vi "Main_16B_X1.vi"() -> ()   [LabVIEW 2024]
uses:
  Cluster_Deer Score and Pose and Set.ctl
  Cluster_Deer Pose.ctl
  Utility/Universal Utility/TypeDefs_Utility/Cluster_Row-Column.ctl
  Utility/Universal Utility/TypeDefs_Utility/ENUM_4 Directions U-D-L-R.ctl
  8beb7c92-1c82-4182-b844-b29be1e81950.vi
  <vilib>/Utility/error.llb/Trim Whitespace.vi
  <vilib>/Utility/error.llb/Trim Whitespace One-Sided.vi
panel:
  out "size(s)":i32
  out "Answer":i32
  out "sorted array":T1[](array[typedef])
  in  "Tab Control":enum32{"Example ", "Eample 2", "Puzzle"}(tab)
  in  "Example":string="###############\n#.......#....E#\n#.#.###.#.###.#\n#.....#.#...#.#\n#.###.#####.#.#\n#.#.#.......#.#\n#.#.#####.###.#\n#...........#.#\n###.#.#####.#.#\n#...#.....#.#.#\n#.#.#.###.#.#.#\n#.....#...#.#.#\n#.###.#.#.#.#.#\n#S..#.....#...#\n###############"
  in  "Example 2":string="#################\n#...#...#...#..E#\n#.#.#.#.#.#.#.#.#\n#.#.#.#...#...#.#\n#.#.#.#.###.#.#.#\n#...#.#.#.....#.#\n#.#.#.#.#.#####.#\n#.#...#.#.#.....#\n#.#.#####.#.###.#\n#.#.#.......#...#\n#.#.###.#####.###\n#.#.#...#.....#.#\n#.#.#.#####.###.#\n#.#.#.........#.#\n#.#.#.#########.#\n#S#.............#\n#################"
  in  "Puzzle":string="#############################################################################################################################################\n#.....#.....#.....#.........#.....#.......#...#.........#.....#.....#...........#...#.............#.....#.....#...........#.....#..........E#\n#.###.#.###.#.###.#####.#.#.#.###.#.#####.#.#.#.###.###.#.#.###.###.#.#######.###.#.#.###.#######.###.#.###.###.###.#####.#.###.#.#####.###.#\n#.#.....#.#.#.#.....................#.....#.....#...#...#.#.......#.#...#...#.....#.#.#.#.....#.#.....#...#...#.#.#...#.....#...#...#...#...#\n#.#######.#.#.#######.###.#.###.###.#.#.###.#####.#.#.###.#######.#.###.#.#.#######.#.#.#####.#.#########.###.#.#.###.#######.###.###.###.###\n#...........................#...#...#.#.#...........#.#...#.#...#.#.#...#.#.....#...........................#.......#...#...#...#.#...#.....#\n#.###.#.#.#.###.#.#.#######.#####.#.#.#.#.###.###.#.#.#.###.#.#.###.#.###.#####.#.#.#####.#.###.###.#######.###########.#.#.###.#.#.###.#####\n#.#...#.#.#.#...#.#...#...........#.........................#.#...#.#.#...#...#.#.#...#...#.#.......#.#...#.........#...#.#.#...#.#.#...#...#\n#.#.###.#.#.#.###.#####.#####.#####.#.###.###.#.#.#.#########.###.#.#.#####.#.#.#.###.#.###.#.#######.#.#.#########.#.#####.#.###.#.#####.#.#\n#.#...#.#...#.#.......#.#.....#...#.#...#.....#...#...........#.#.#.........#...#...............................#...#...#...#.#...#...#...#.#\n#.###.#.#####.#######.#.#.#######.#.#.#.#######.#.#.#.###.#####.#.###.#.#######.#######.#.#.#####.###.#.#.#.#.#.#.#####.#.###.#######.#.###.#\n#.#.#.#.......#.......#...#.#.....#.#.#.......#.#.#.#.#...#...#.....#.#.....#...#.........#.#...#.....#.................#.......#...#...#...#\n#.#.#.#########.#####.#####.#.#.###.#.#.#######.#.#.#.#.###.#.#####.#.#####.#.#########.#.#.###.###.###.#.#.###.#.#.#.#########.#.#.#####.#.#\n#...#.#.........#.......#...#.#.....#.#.....#...#...........................#.........#...#.............#.#...#...#.#.....#...#...#.......#.#\n###.#.#.#####.###.###.#.#.#.#.#######.#####.#.###.###.###.#.#####.#.#.###########.###.#.#####.#.#.###.###.###.#####.#####.#.#.#############.#\n#...#.#.....#.....#...#...#.......#.....#...#.#.....#.#...#.#...#.#...#.............#.#...#...#.....#...#...#.#...#.#...#...#.#.............#\n#.#.#.#####.#######.#.###########.#.#####.#.#.#.###.#.#####.#.###.###.#######.#.#.###.###.#.#######.#.#####.#.#.#.#.#.#.#####.###.#.#######.#\n#...#...#.#...#.....#.........#...#...#...#.#.#.#...#.......#...#.#.#.#.....#.#...#.......#.......#.#.#.....#.#.#.....#.....#...#.#.....#...#\n#.#####.#.###.#####.#########.#.###.#.#.###.#.###.#############.#.#.#.#.###.#.#.###.###########.#.#.#.#.#####.#.###########.###.#####.#.#.###\n#.#.....#...#.....#.........#...#.#...#...#.#...#...#...........#.#...#.#.#.#.#.....#.#.......#.#.....#.#...#.#...#...#.....#.#.....#.#...#.#\n#.#.#.#####.###.#.#####.#########.###.###.#.###.#.#.#.###.#####.#.#.###.#.#.#####.###.#.#####.#########.#.#.#.#.###.#.#.#####.#####.#.#####.#\n#.#.#.#...#.....#.....#...............#...#.#.#.#...#.#.#...#.#.#.#.#...#.#.....#.....#.#...#.....#.....#.#.#.#.#...#.#.#.....#.....#.#.....#\n#.#.###.#.#.#########.#.###############.###.#.#.#.###.#.###.#.#.#.#.#.###.#####.#######.#.#######.#.#######.#.###.###.#.#.#.###.#####.#.###.#\n#.#.....#.#.......#...#...#...........#...#...#.#...#.#...#.#.#.#.#...#.........#.......#.......#.#.#.......#.....#.#.#.#.#.#.......#.#.#...#\n#.#######.#####.###.#####.#.#.#######.###.#####.###.#.#.#.#.#.#.#.#############.#.#########.###.#.#.###.###########.#.#.#.###.###.#.#.#.###.#\n#.#.....#.#...#.#...#...#.#.#.#.....#.#.#.....#...#.....#...#.#.#...#.........#...........#...#.....#...#.........#...#.#...#.#...#.#.#...#.#\n#.#.#####.#.#.#.#.###.###.###.#.###.#.#.#####.###.###.#####.#.#.###.#.#######.#.#######.#.###########.###.#######.#.###.#.#.#.###.###.###.#.#\n#...#.....#.#...#...#...#.....#...#.........#.......#.#...#.#.....#.........#.#.#.....#.#.......#.....#.....#...#.#.#...#.#.#...#...#.....#.#\n###.#.#####.###.###.###.#.###############.#######.#.###.#.#.#.#############.#.#.#.###.#########.#.#####.#####.#.#.#.###.###.###.#.#.#######.#\n#.#.#.#.......#.#.#...#...#.............#.#.......#...#.#...#.#...........#.#.#...#.#...........#.........#...#...#...#.....#...#...........#\n#.#.#.#.#.#.#.#.#.###.#.#.#.#####.#.###.###.#####.###.#.#####.#.#.#######.###.#.###.#############.#########.#.#######.#.#####.###.#.###.#####\n#...#.#.#...#.#.....#.#...#.......#.#...#...#...#...#...#...#.#...#.....#.#...#...........#.....#...#.......#.#.....#...#.....#...#...#.#...#\n#.###.#.#####.###.###.#.#######.#.#.#.###.###.#####.#####.###.#.#.#.###.#.#.###.###.#######.###.###.#.#######.#.###.#.#.#.###.#####.#.#.###.#\n#...#.#.#...#.#.#.#...#...#.#...#...#.#...#...........#.....#...#.#...#.#...#...#.#.#.......#.#...#.#.......#.....#...#.#...#.#.....#.#...#.#\n###.#.###.#.#.#.#.#.#####.#.#.#######.#.###.#########.#####.###.#.###.#.#####.###.#.#.#######.###.#.#######.#####.#########.###.###.#.###.#.#\n#...#.#...#...#...#...#.....#...#...#.#...#.....#...#.....#.....#...#.#...#.......#.#.....#...#...#.#.....#.......#...........#...#.#.......#\n#####.#.#.###.#######.#.#######.#.###.#.#.#######.#.#####.#######.#.###.#.#.#######.#####.#.#.#.###.#####.#########.#.###.#.#.#.###.#######.#\n#...#.#.#.....#...#...#.#.......#.....#.#.......#.#...#...#.....#.#...#.#.#...........#.#.#.#.#...#.#.....#...#.....#.#.#.#.#.......#...#...#\n#.#.#.#.#.#####.#.#.#####.###.###.#####.#.#####.#.###.###.#.###.#####.#.#####.#.#####.#.#.###.###.#.#.###.###.#.###.#.#.#.#######.#.#.#.#.###\n#...............#.........#...........#.#.....#.#...#...#...#...#.....#.......#.#...#.#.#...#...#.....#...#...#.#.....#.#...#.....#...#.#...#\n#.#####.#.#################.#########.###.###.#.###.###.#####.###.###.#.#.#####.#.#.#.#.###.#.#.#####.#.###.#.#.#.#####.###.#.###.#.###.###.#\n#...#.#...#...#...#.....#...#.......#...#...#...#...#.#.....#.#...#.#.........#.#...#.......#.#.......#.#...#.#.#.........#.#.............#.#\n###.#.###.#.#.#.#.###.###.###.#####.###.###.###.#.###.#####.#.#.###.#.#.#######.#.###.#####.###.#######.###.###.#.#####.###.#.#####.#.###.#.#\n#...#...#...#.#.#...#.......#.#...#.#...#.....#.#.#...#.....#...#.....#.........#.....#.....#...#.....#...#.....#.....#.....#.#.......#.#.#.#\n#.###.#.#.###.#.###.#.#.#####.#.#.#.###.#.#.#.#.#.#.#.#.#########.#####.#########.#####.#####.###.###.###.#.#########.#.#####.#.###.###.#.###\n#...#.#.......#...#...#.#.....#.#.#...#...#.....#.#.#.#.#...#.......#...#.........#.....#.....#...#.#...#.#.......#.#.#...#.....#.......#...#\n#.#.#####.#.#.#.#.###.###.#####.#.###.#####.#####.#.#.#.#.###.#######.###.###.#.###.#######.#.#.###.###.#.#######.#.#.###.#.#######.#.#.###.#\n#.#.......#...#...#.#...#.....#.....#.#...#...#...#.#.#.#.....#.......#...#...#...#.#.......#...#.....#...#.#.......#.#...#.#.......#.#.#.#.#\n#.#######.###.#.###.###.#####.#.###.#.#.#.###.#.#####.#.#######.###########.#.#####.###.#####.#.#.#.#######.#.#####.#.#.###.#####.#.#.#.#.#.#\n#.....#.#.............#.#...#...#...#.#.#...#.#...#...#.#.....#...#...#...#...#...#.....#.....#.#.#.#...#...#.#...#.#.#.#...#.....#.#.#...#.#\n#.###.#.#.###.#######.#.#.#.#.#.#####.#.###.#.###.#.#.#.#.###.###.#.#.#.#.#.#.#.#.#######.#####.#.###.#.#.#.#.#.#.###.#.#.#.#.#####.#.#####.#\n#.............#...#...#...#.....#.....#...#.........#.#...#.#.#...#.#...#...#...#...#.....#.....#.....#...#.#.#.#...#.#...#...#...#...#.....#\n#.###########.#.#.###############.#######.#############.###.#.#.#.#.###############.#.#.#.#.#####.#########.#.#.#.#.#.###.#####.###.#.#.###.#\n#.#.....#.....#.#...........#...#.......#.#...#.......#.....#.#.#.#.#...#.....#...#...#.#.#.....#.........#...#.#.#...#.........#.....#.#.#.#\n###.###.#.#.#.#.###.#######.#.#.#######.#.#.###.#####.#####.#.#.#.#.###.#.#.#.#.#.#####.#.#####.#########.#####.#.#####.###.###.#.#####.#.#.#\n#...#...#.#.....#.......#.#...#...#...#.#.....#.#...#.....#.#.#.#.#...#.#.#.#...#.#...#.#.#.....#...#...........#...#...#.....#.#.#.....#.#.#\n#.#####.#.###.###.#####.#.#######.#.#.#.#.#.#.#.#.#.#####.###.#.#####.#.#.#.#####.###.#.#.#.#####.#.#######.#######.#.###.#####.#.#.#####.#.#\n#.....#.#.......#.#...#.....#...#...#.#.#.#...#.#.#.....#...#.#.......#...#.#.........#.#.#.#.....#...#...#.#.....#...#...#...#...#...#.#...#\n#.###.#.#######.#.#.#.#.#####.#.###.#.#.#.#.###.#.#####.#.#.#.###.#########.#.#######.#.#.#.###.#.###.#.#.#.#.###.#.#####.#.#.#.#####.#.#.###\n#...#.#.#...#...#.#.#...#...#.#.............#...#.#...#.....#...#...........#...#.....#.#.#...#.#...#...#.#.....#.#.#...#.#.#.#.....#.#.....#\n#####.#.#.#.#.###.#######.#.#.#############.#.###.###.#########.###############.#.#####.#.###.#.###.###.#.#####.#.#.#.#.###.#.###.###.#####.#\n#.....#...#.#.#.#.........#...#.#...#.......#...#...#.....#.....#.........#...#.#.#.....#.#...#.#...#...#...#.#.#.#...#.....#...#.#...#...#.#\n#.#####.###.#.#.#.#.###########.#.#.#.#########.###.#.###.#.#.###.#######.#.#.#.#.#.#####.#.#####.###.#.###.#.#.#.#############.#.#.#.#.#.#.#\n#.............#.#.....#.........#.#...#.....#.#...#...#.#.#.#...#...#...#...#.#.........#.#.......#.........#...#.....#.........#.#.#.#.#.#.#\n#.###########.#.#####.###.#####.#.#####.#.#.#.###.#####.#.#.###.#.###.#.#.###.#.#######.#######.#.#########.#.#######.#########.###.###.#.#.#\n#.#.......#...#.....#.#...#.#...#.#...#.#.......#.#...#...#.#...#.#...#.#.#...#.#.....#.......#.#.#...#...#.#.......#...#.....#.....#...#.#.#\n#.#.#####.#.#.#.#.#.#.#.###.#.#.#.#.#.#.#.#.#####.#.#.#.#####.###.#.###.###.###.###.#####.#####.#.#.#.#.#.#.###########.#.###.#.#####.###.#.#\n#...#...#.#.#.#.#.#.#.#.#.......#...#.#.#.#.#.....#.#.#.......#...#.#.....#.#.......#.....#.....#...#...#.#...........#...#...#.#.....#.#.#.#\n#.###.#.#.###.#.#.###.#.#.###########.#.#.###.#####.#.#######.#.###.#####.#.#########.###.#.#########.###.###########.###.#.###.#.#####.#.###\n#.....#.#...#...#.....#.#.#.........#.#.#.#...#.....#.....#...#.........#.#.........#...#...........#...#.#.........#...#.#.#.#.#.#.........#\n#######.###.#.#####.###.###.#######.#.###.#.###.#######.#.#.#####.#####.#.#.#######.#.#.###########.#####.#.###.#######.#.#.#.#.#.#.###.###.#\n#.....#.#...#...#...#.#.............#.....#.#.....#...#.#.#.....#.#...#.#.#.#.#...#.#.....................#...#...#.....#.#.#...#.#.#...#.#.#\n#.###.###.#.###.#.#.#.#.###########.#####.#.#####.#.###.#.#####.#.###.###.#.#.#.#.#.#########.###########.#######.#.#####.#.#.###.###.#.#.#.#\n#.#.#...#.....#...#.#...#...........#.....#...#...#...#.#.....#.#.....#...#...#.#.#.....#...#...#...#.....#.....#.#.....#.#.#.#...#...#.#.#.#\n#.#.###.###.#.#####.#####.#######.###.#.#.###.#.#####.#.#######.###.#.#.#######.#.###.#.#.#.###.#.#.#######.###.#.#####.###.#.#.###.###.#.#.#\n#.#.........#...#.#...#...#.....#.#...#.....#.#.......#...#...#.#.#.#.#.........#...#.#.#.#.#...#.#...#.....#...#...#...#...#.#...#.#...#.#.#\n#.#########.###.#.###.#.#.#.###.###.#########.###########.#.#.#.#.#.#.###########.#.#.#.#.#.###.#.###.#.#####.#####.#.###.###.###.#.#.###.#.#\n#.#.....#.#.#...#.....#.#.#...#...#.....#...#.#.........#.....#...#...#.......#...#.#.#.......#.#.#.#...#.....#...#...#...#.....#...#.#...#.#\n#.#.###.#.#.#.###.#.###.#.###.###.###.#.#.#.#.#.#######.#####.#.#.###.#.#####.#.#.#.###.#####.###.#.#####.#####.#.#.###.#####.#######.#.#.#.#\n#...#...#...#...#...#...#...#.#.#.......#.#.#.#.#.....#.#.....#.#.#.#.#.....#...#.#...#.#...............#.....#.#.#.....#...................#\n#####.###.#.#.#.#.#####.#.###.#.#####.#.#.#.#.#.#.###.#.#.###.#.#.#.#.#.###.###.#####.###.#.###########.#####.#.#.#######.###############.#.#\n#.....#.#...#.#...#.....#.#...#.........#.#...#.......#...#.#...#...#.#...#...#.#...#.....#.....#...#...#.#...#.#...#.....#.......#...#...#.#\n#.#####.###.#.#.###.#.#####.###.#####.###.#####.#.#.###.###.###.#.###.###.###.###.#.###########.#.#.#.###.#.###.#.#.#.###########.#.#.###.#.#\n#.#...#...#...#.#.#.#.....#.#...#.......#.#.....#.#.......#.....#.....#.#...#.....#.......#.....#.#.........#.....#...............#.#...#.#.#\n#.#.#.#.#.#.###.#.#.#####.#.###.#.#####.#.#.#####.#.###.###.#####.#.###.###.#############.#.#############.#.#.#####.#########.#.###.###.###.#\n#...#.#.#.....#.#...#.....#...#.....#...#.#.#.#...#.#.#.....#.....#.#.........#.......#.............#...#.#...#.........#...#.#.#...#.#.....#\n#.###.#####.###.#.###.#######.#######.#.#.#.#.#.###.#.#######.#####.#.#######.#.#####.#.#.#########.#.#.#.###.#.###.#####.#.#.#.#.###.#######\n#.#.#.....#.....#...#.......#.#.....#...#.#...#...#...#.......#.#...#...#...#.#...#.....#.......#...#.#.#.#...#.....#.....#.#.#.#...#.......#\n#.#.#####.#.#.###.#########.#.#.###.###.#.###.###.###.#.#######.#.#######.#.#####.###############.###.#.#.#.#####.#.#.#####.#.#.###.#.###.#.#\n#.#.....#...#.#...#.......#.#.#.#.#...#.#.#.....#...............#.#.....#.#.......#.....#.......#.#...#.....#...#.#.#.#.#...#.#.#...#...#.#.#\n#.#.#.#.###.#.###.#.#####.#.#.#.#.###.#.#.###.#####.#####.#####.#.###.#.#.#.#####.#.###.#.#####.#.#.#########.#.#.#.#.#.#.#.#.#.#.###.#.#.###\n#.#.#.#.........#.#...#.....#.#.#...#.#.#...#.#...#.#...#.#...#.#.#...#...#.....#.#...#...#.#...#.#.#.....#...#.#.#.#.#.#.......#...#...#...#\n#.#.###.#######.#####.#######.#.#.#.#.#.###.###.#.###.#.###.#.#.#.#.#######.###.#####.#####.#.###.#.#.###.#.###.#.#.#.#.###########.#.#####.#\n#...........#.#.......#.....#.#.#.#.#.#...#.....#...#...#...#.#.#.#.#...#...#.#.....#.....#.#...#.....#.#.#.#.......#.#.#...........#...#...#\n#.###.#.###.#.#.#.###.#.###.#.#.#.#.#.#.###########.#.#.#.#.#.###.#.#.#.#.###.#####.#####.#.###.#######.#.#.#######.#.#.#.###########.#.#.#.#\n#...............#.#...#.#.#...#.#.#...#.........#.#...#...#.#.....#.#.#...#.......#.......#...#.......#...#.......#.#...#.......#.....#...#.#\n#####.#.#####.###.#.###.#.#####.###.#####.#####.#.#########.#######.#.#######.#.#.###########.#.#######.#########.###.###.#.###.#.###.#####.#\n#...#.#...#.......#.#...#.........#.....#...#.#...#...........#.....#.....#...#.#.#...........#...#...#.#.......#.....#...#.#.....#.......#.#\n#.###.#.#.#######.###.###.#######.#.###.###.#.###.#.#####.#.#.###.#.#####.#.###.#.#.###.#.#######.#.#.#.#.#####.#####.#.###.#######.#.###.#.#\n#...#...#.......#.#...#.......#...#...#.....#.#...#...#.#...#...#.#.....#.#...#.#.#.#.#.#.......#...#.#...#...#.......#.......#.......#.#.#.#\n#.#.###.#######.#.#.#####.#####.###.#########.#.#####.#.###.###.#.###.###.#.#.#.#.#.#.#.#.#####.#####.#####.#.#####.#.#.#####.#.#####.#.#.###\n#.#...#.....#...#.#.....#.......#.....#.......#.#...#.....#.#...#...#.....#.#...#.....#.......#.#.........#.#.......#.#.....#...........#...#\n#.#.#.#.###.#.###.#####.###.#####.###.#.#####.#.#.#####.###.#.###.#####.#.#.#.#.#.###########.#.#.#######.#.###.#.###.#####.###.#.#.#.#####.#\n#.#.#.#.....#...#.....#.#...#.....#...#.#...#...#.....#.#...#...#.#.....#.#.#.#.#...#.....#.#.#.#.......#.#...#.#.#.......#.................#\n#.#.###.#######.#.#####.#.###.#####.#.#.#.###########.#.#.#####.###.#####.###.#.#####.###.#.#.#.#######.#.#.#.#.#.###########.#.#.#####.#.#.#\n#.#...#.......#.#.#.........#.#...#.#.#.#...........#.#.#.#...#...#.....#.....#.......#.......#...#.....#.#.#.#.#.............#.#.#...#...#.#\n#.###.#.###.#.#.###.#######.#.#.###.#.#.#.#####.###.#.#.#.###.###.#.###.#####.#########.#########.#.#####.###.#.###############.#.#.#.#####.#\n#...#...#.....#...#...#.....#...#...#.#.#.#.#...#.......#...#.....#.#.#.......#...#...#.#.....#...#.#...#.....#.....#.......#...#...#.#.#...#\n###.#.###.#.#####.###.#.#######.#.#####.#.#.#.#########.###.#.#####.#.#########.#.#.#.#.#.###.#.###.#.#.#######.#.#.#.#####.#.#####.#.#.#.###\n#...#.#...#.........#...#.....#.#...#...#.#.#.............#.#.....#.....#.......#...#.#...#.#.#.#...#.#.......#.#.#.#.....#.......#.#.......#\n#.###.#.###.#######.#######.#.#####.#.###.#.#############.#.#####.#######.###########.#####.#.#.#.###.#####.###.#.#.###.#########.#.#.#.#.#.#\n#.................#...#.....#.....#.#.#.#...#.......#...#.#.....#.....#...#.........#...#...#...#...#...#...#...#.#.....#.....#.#...#.#.#.#.#\n###.#####.#.#.###.###.###.#######.#.#.#.#.###.#####.#.#.#.#####.#####.#.###.###.#######.#.#.#.#.###.###.#.###.###.#######.###.#.###.#.#.#.#.#\n#.#.......#.....#...#...#.#.....#...#.....#...#...#.#...#.....#...#.....#.#.#.#.........#.#...#...#.#...#.#...#...#...#...#...#.....#.#.....#\n#.###.#####.###.###.###.#.#.###.###.#.#####.###.#.#.#.#.#####.###.#######.#.#.###########.#.#####.#.#.###.#.###.###.#.#.###.###.###.#.#.#####\n#...#.#...........#.#.....#...#.#...#.......#.....#...#.#.....#...#...#...............#...#.......#.#.#.#.#.#.#...#.#...#.#...#.#.....#.#...#\n#.###.#.###.#######.#######.###.#.#############.#.#####.#######.#.#.#.#######.#######.#.###########.#.#.#.#.#.#.###.#####.###.###.#.#####.#.#\n#.....#...#.....#...#.......#...#.....#.........#.....#.#.......#.#.#.....#.....#.....#.....#.......#.#.#...#...#.....#.....#...#...#.....#.#\n#########.#.#.#.#.###.#.#.###.###.#####.#.#####.#######.#.#########.#####.#.#.###.#######.###.#####.#.#.#########.#.#.#.###.###.###.#.#####.#\n#.........#...#.#.....#.#...#...#.#.....#...........#...#.#...#...#.#...#.#.#.......#.....#...#...#...#.........#...#.....#...#...#.....#...#\n#.#########.#.#.#.#####.###.###.#.#.#.#############.#.###.#.#.#.#.#.###.#.#########.#.#.###.#.#.#.###.#####.###.#.#.#.###.###.###.#.#.###.#.#\n#.#.........#...#.....#.#...#.#...#...#.........#.....#.#...#.#.#...#...#.........#...#...#.#.#.#...#.#.....#...#.#.#.......#...#.........#.#\n#.###.#####.#.#########.###.#.#######.#.#######.#.###.#.#.###.#.#####.#######.###.#######.#.###.###.#.#.#####.#####.#######.#.#.###.#######.#\n#...#.#.....#...#.....#...#...#.....#.#.......#.#.....#...#...#...#...#.......#.#...#.#.....#...#...#.#...#.#.....#.......#.#.#.........#.#.#\n###.###.###.###.#.###.###.###.#####.#.#########.#######.###.#####.###.#.#.###.#.###.#.#.#####.###.###.###.#.#####.#.#####.###.#.###.###.#.#.#\n#...#...#.#...#...#.#.....#...#.....#.........#.......#.#.#.....#...#...#...#...#...#.....#...#...#.#.....#...#...#.#.....#...#.#.....#...#.#\n#.###.###.###.#####.#######.###.###.#######.#.#.###.###.#.#####.###.###.###.#####.#.#####.#.###.###.#######.###.###.#.#####.###.#.#.#.#####.#\n#...........#.#.....#.#.....#...#.#.#.#.......#.......#.#.....#...........#.....#.#.#.........#...#...#.....#...#...#.......................#\n#.#####.###.#.#.###.#.#.#######.#.#.#.#.#######.#####.#.#####.#########.#.#####.#.###.###.#######.#.#.#.###.#.#.#####.#.#.#.#####.#.###.#.###\n#.......#...#.#.#.....#...#.....#.#...#.#.....#...#.#.......#...#...#...#.#.....#...........#...#.#.#.#.#.#...#.......#.#.#.......#...#.#.#.#\n#########.###.#.#####.###.#.#####.###.#.###.#.###.#.#######.###.#.#.#.#.#.#.###.###########.#.#.#.#.#.#.#.#####.#######.#.###########.#.#.#.#\n#.....#...#...#.....#...#.#.#.....#...#...#.#.......#.....#.....#.#.#.......#.....#.....#...#.#...#.#.#.#...#.....#.....#.#...........#...#.#\n#.#####.###.#####.#.###.#.#.#####.#.#####.#.#######.#.###.#######.#.###.#########.#.###.###.#.#######.#.#.#.###.#.#.###.#.#.###.#####.#####.#\n#.#.......#.#...#.#.#...#...#...#.......#.#.#...#.#.#.#...#.......#...#...#.....#.#.#.#.......#.......#...#...#...#.#.#.#.#.................#\n#.#.#######.#.#.###.#####.###.#.#####.###.###.#.#.#.#.###.#.#########.#.#.#.###.###.#.#####.###.#####.#######.#.###.#.#.#.#.#.###.#.#####.#.#\n#...#.....#.#.#...#.......#...#.....#.#...#...#.#...#...#...#.......#...#.#...#.....#.....#.....#.....#.......#.#.....#.#.#.#...#.#.....#.#.#\n#.###.#.#.#.#.###.###.#####.#######.###.###.###.#.#####.#.#####.#######.#.###.#######.###.#.###.#######.#######.#.#####.#.#####.#.###.#.#.#.#\n#.#...#.#.................#.......#.....#...#...#.#...#.......#.#...#...#.#...#.....#.#.#.#.#.#.....................#...#.....#.#...#.#.#.#.#\n#.###.#.#####.#.###.###.#.#######.#.#######.#.#####.#.###.###.#.#.#.#.#.###.###.###.#.#.#.#.#.###.#.#.#.#.###.#.#.#.#.#######.#.###.#.###.#.#\n#S....#...........#.....#...................#.......#.........#...#.........#.....#.....#.......#...#.....#.....#...#...........#...#.......#\n#############################################################################################################################################"
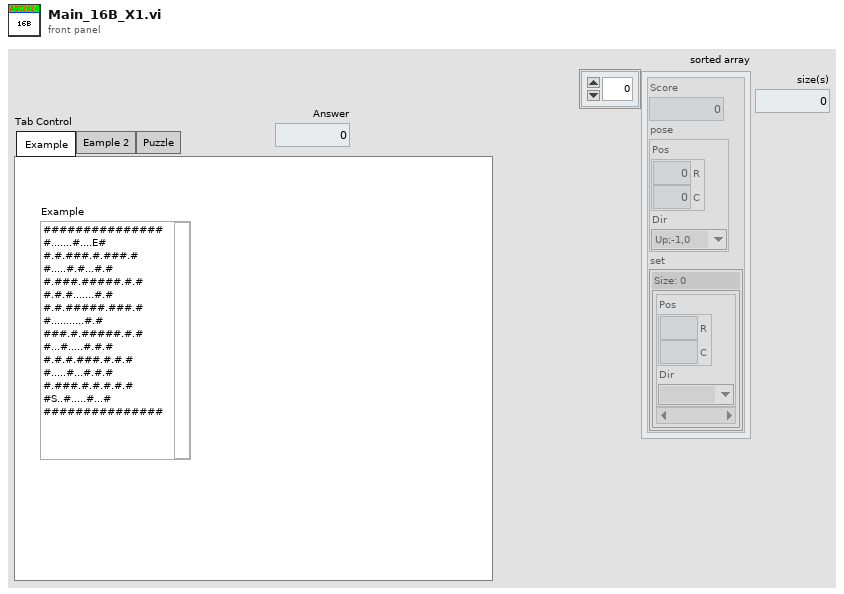
[diagram p1: front panel]
types:
  T1 = typedef "Cluster_Deer Score and Pose and Set.ctl" = cluster{"Score":u32, "pose":T2, "set":set{T2}}
  T2 = typedef "Cluster_Deer Pose.ctl" = cluster{"Pos":T3, "Dir":T4}
  T3 = typedef "Cluster_Row-Column.ctl" = cluster{"R":i32, "C":i32}
  T4 = typedef "ENUM_4 Directions U-D-L-R.ctl" = enum16{"Up;-1,0", "Right;0,1", "Down;1,0", "Left;0,-1"}
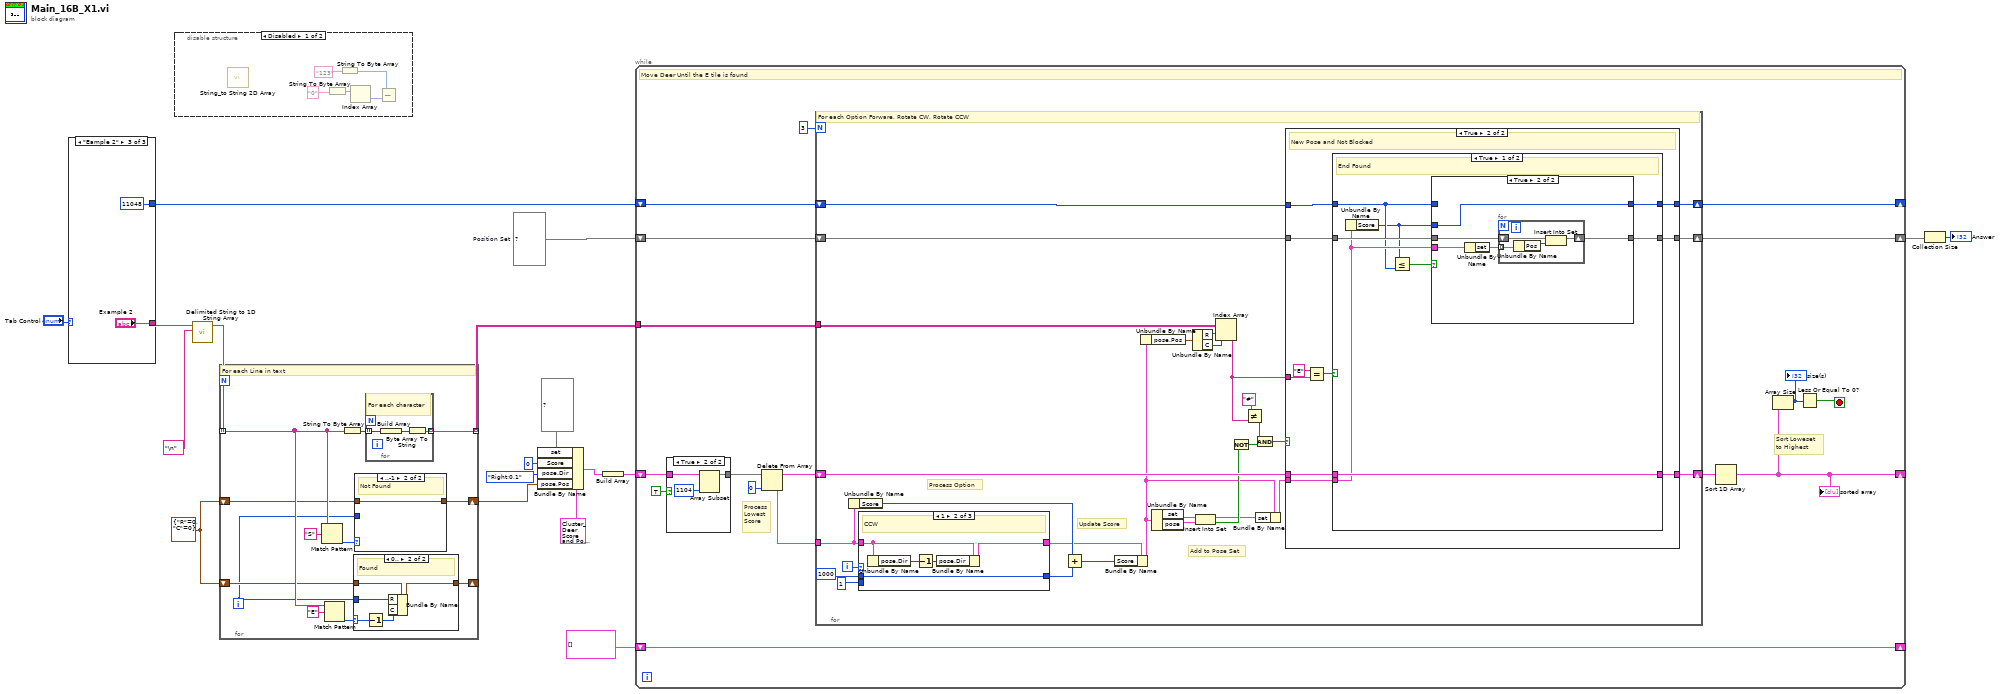
[diagram p0: block diagram]
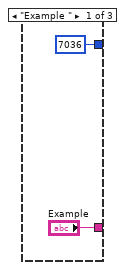
[diagram p2: hidden frame]
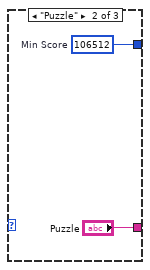
[diagram p3: hidden frame]
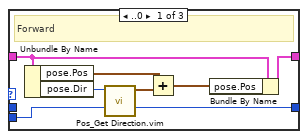
[diagram p5: hidden frame]
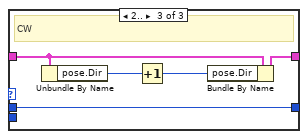
[diagram p6: hidden frame]
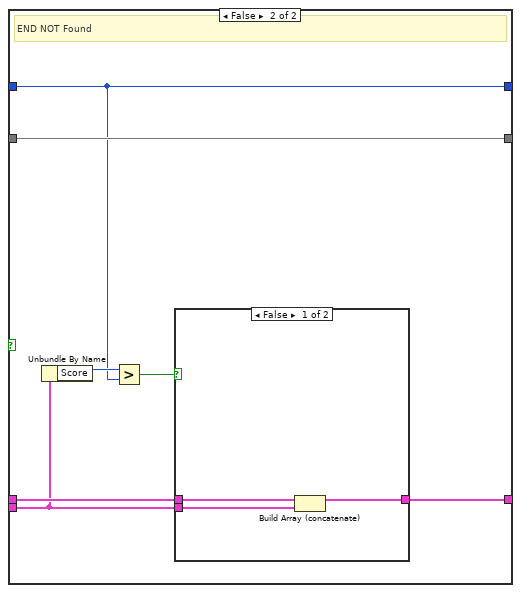
[diagram p9: hidden frame]
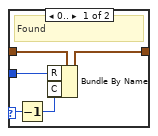
[diagram p13: hidden frame]
diagram:
  w6 = set{T3} {}  # Position Set
  w16 = T3 {"R"=0, "C"=0} ("Position")
  n1 = case shown="\"Eample 2\"" "Tab Control" {
    tunnel: ["Example" "Puzzle" "Example 2"] -> w8
    tunnel: [u32 7036 ("Min Score") w21 u32 11048 ("Min Score")] -> w1
    frame "Example " {
    }
    frame "Puzzle" {
      w21 = u32 106512  # Min Score
    }
    frame "Eample 2" {
    }
  }
  n2 = disable-structure shown="Disabled" {
    frame Disabled {
      n3 = call "String_to String 2D Array.vi"() -> ()  [unwired: 11 in, 1 out]
      n4 = String To Byte Array(string="0") -> (unsigned byte array=w27:u8[])
      n5 = String To Byte Array(string="123") -> (unsigned byte array=w25:u8[])
      n6 = Index Array(array=w27) -> (element=w26:u8)  [unwired: 1 in]
      n7 = Subtract(x=w25, y=w26) -> ()  [unwired: 1 out]
    }
    frame Enabled {
    }
  }
  n8 = call <vilib>:"Delimited String to 1D String Array.vi"("delimiter"="\n" ("delimiter (Tab)"), "delimited string"=w8) -> ("string array"=w17:string[])  [unwired: 9 in]
  n9 = for {
    tunnel: w17 -> [w40] mode=indexing
    shift-right: [w32] -> w7
    shift-left: w16 -> [w35]
    shift-right: [w31] -> _
    shift-left: w16 -> [w34]
    tunnel: [w30] -> w13 mode=indexing
    i -> [w33]
    # "For each Line in text"
    n10 = Match Pattern(string=w40, regular expression="S") -> (offset past match=w36:i32)  [unwired: 1 in, 3 out]
    n11 = Match Pattern(string=w40, regular expression="E") -> (offset past match=w37:i32)  [unwired: 1 in, 3 out]
    n12 = String To Byte Array(string=w40) -> (unsigned byte array=w41:u8[])
    n13 = case shown="0.." w37 {
      selector: w37 -> [_ w45]
      tunnel: w34 -> [w42 w47]
      tunnel: w33 -> [_ w46]
      tunnel: [w42 w44] -> w31
      frame ..-1 {
        # "Not Found"
      }
      frame 0.. {
        # "Found"
        n14 = Decrement(x=w45) -> (x-1=w43:i32)
        n15 = Bundle By Name(cluster=w47, "R"=w46, "C"=w43) -> (w44:T3)
      }
    }
    n16 = case shown="..-1" w36 {
      selector: w36 -> [w50 _]
      tunnel: w35 -> [w52 w53]
      tunnel: w33 -> [w51 _]
      tunnel: [w49 w53] -> w32
      frame 0.. {
        # "Found"
        n17 = Decrement(x=w50) -> (x-1=w48:i32)
        n18 = Bundle By Name(cluster=w52, "R"=w51, "C"=w48) -> (w49:T3)
      }
      frame ..-1 {
        # "Not Found"
      }
    }
    n19 = for {
      tunnel: w41 -> [w56] mode=indexing
      tunnel: [w54] -> w30 mode=indexing
      # "For each character"
      n20 = Build Array(w56) -> (w55:u8[])
      n21 = Byte Array To String(unsigned byte array=w55) -> (string=w54:string)
    }
  }
  n22 = Bundle By Name(cluster=T1 {"Score"=0, "pose"={"Pos"={"R"=0, "C"=0}, "Dir"=enum."Up;-1,0"}, "set"={}} ("Dear pos and direction"), "set"=set{T2} {}, "Score"=u32 0, "pose.Dir"=ENUM_4_Directions_U-D-L-R."Right;0,1" ("Direction"), "pose.Pos"=w7) -> (w11:T1)
  n23 = Build Array(w11) -> (w10:T1[])
  n24 = while {
    shift-right: [w63] -> _
    shift-left: w10 -> [w59]
    tunnel: w13 -> [w72]
    shift-right: [w66] -> w5
    shift-left: w6 -> [w67]
    shift-right: [w64] -> _
    shift-left: w1 -> [w65]
    shift-right: [w60] -> _
    shift-left: T1[] [] ("appended array") -> [w60]
    stop <- w61 stop-if-true
    # "Sort Loweset \nto Highest"
    # "Process\nLowest \nScore"
    # "Move Deer Until the E tile is found"
    n25 = case shown="True" TRUE {
      tunnel: w59 -> [w74 w77]
      tunnel: [w74 w76] -> w58
      frame False {
      }
      frame True {
        n26 = Array Subset(array=w77, length=1104) -> (w76:T1[])  [unwired: 1 in]
      }
    }
    n27 = Delete From Array(array=w58, index=0) -> (deleted portion=w70:T1, array with subset deleted=w69:T1[])  [unwired: 1 in]
    n28 = for {
      N: 3 -> [_]
      tunnel: w70 -> [w98]
      tunnel: w72 -> [w105]
      shift-right: [w99] -> w68
      shift-left: w69 -> [w100]
      shift-right: [w82] -> w66
      shift-left: w67 -> [w84]
      shift-right: [w80] -> w64
      shift-left: w65 -> [w81]
      i -> [w106]
      # "Add to Pose Set"
      # "Update Score"
      # "Process Option"
      # "For each Option Forware, Rotate CW, Rotate CCW"
      n29 = Unbundle By Name(w98) -> ("Score"=w97:u32)
      n30 = case shown="1" w106 {
        tunnel: w98 -> [w109 w115 w120]
        tunnel: [w107 w116 w121] -> w96
        tunnel: [w113 w114 w119] -> w78
        tunnel: u32 1000 -> [_ w114 w119]
        tunnel: u32 1 -> [w113 _ _]
        frame ..0 {
          # "Forward"
          n31 = Unbundle By Name(w109) -> ("pose.Pos"=w110:T3, "pose.Dir"=w112:T4)
          n32 = call "Pos_Get Direction.vim"("Direction"=w112) -> ("Position"=w111:T3)  [unwired: 10 in]
          n33 = Add(x=w110, y=w111) -> (x+y=w108:T3)
          n34 = Bundle By Name(cluster=w109, "pose.Pos"=w108) -> (w107:T1)
        }
        frame 1 {
          # "CCW"
          n35 = Unbundle By Name(w115) -> ("pose.Dir"=w118:T4)
          n36 = Decrement(x=w118) -> (x-1=w117:T4)
          n37 = Bundle By Name(cluster=w115, "pose.Dir"=w117) -> (w116:T1)
        }
        frame 2.. {
          # "CW"
          n38 = Unbundle By Name(w120) -> ("pose.Dir"=w123:T4)
          n39 = Increment(x=w123) -> (x+1=w122:T4)
          n40 = Bundle By Name(cluster=w120, "pose.Dir"=w122) -> (w121:T1)
        }
      }
      n41 = Add(x=w97, y=w78) -> (x+y=w95:u32)
      n42 = Bundle By Name(cluster=w96, "Score"=w95) -> (w86:T1)
      n43 = Unbundle By Name(w86) -> ("pose.Pos"=w92:T3)
      n44 = Unbundle By Name(w86) -> ("set"=w89:set{T2}, "pose"=w88:T2)
      n45 = Unbundle By Name(w92) -> ("R"=w104:i32, "C"=w103:i32)
      n46 = Insert Into Set(10:w88, 11:w89) -> (2:w91:bool, 3:w87:set{T2})
      n47 = Index Array(array=w105, index (row)=w104, index (col)=w103) -> (element=w83:string)
      n48 = Not(x=w91) -> (.not. x?=w90:bool)
      n49 = Not Equal?(x="#" ("y"), y=w83) -> (x != y?=w94:bool)
      n50 = And(x=w94, y=w90) -> (x .and. y?=w93:bool)
      n51 = Bundle By Name(cluster=w86, "set"=w87) -> (w85:T1)
      n52 = case shown="True" w93 {
        tunnel: w100 -> [w126 w136]
        tunnel: [w126 w135] -> w99
        tunnel: w85 -> [_ w134]
        tunnel: w84 -> [w124 w129]
        tunnel: [w124 w133] -> w82
        tunnel: w83 -> [_ w132]
        tunnel: w81 -> [w125 w128]
        tunnel: [w125 w127] -> w80
        frame False {
          # "Old Pose OR Blocked"
        }
        frame True {
          # "New Pose and Not Blocked"
          n53 = Equal?(x="E" ("y"), y=w132) -> (x = y?=w130:bool)
          n54 = case shown="True" w130 {
            tunnel: w136 -> [w142 w162]
            tunnel: [w142 w160] -> w135
            tunnel: w134 -> [w141 w159]
            tunnel: [w144 w161] -> w133
            tunnel: w129 -> [w143 w161]
            tunnel: w128 -> [w139 w156]
            tunnel: [w137 w156] -> w127
            frame True {
              # "End Found"
              n55 = Unbundle By Name(w141) -> ("Score"=w138:u32)
              n56 = Less Or Equal?(x=w138, y=w139) -> (x <= y?=w140:bool)
              n57 = case shown="True" w140 {
                tunnel: [w145 w151] -> w144
                tunnel: w143 -> [w145 w150]
                tunnel: w141 -> [_ w148]
                tunnel: w139 -> [w146 _]
                tunnel: w138 -> [_ w147]
                tunnel: [w146 w147] -> w137
                frame False {
                }
                frame True {
                  n58 = Unbundle By Name(w148) -> ("set"=w149:set{T2})
                  n59 = for {
                    tunnel: w149 -> [w155] mode=indexing
                    shift-right: [w153] -> w151
                    shift-left: w150 -> [w154]
                    n60 = Unbundle By Name(w155) -> ("Pos"=w152:T3)
                    n61 = Insert Into Set(10:w152, 11:w154) -> (3:w153:set{T3})  [unwired: 1 out]
                  }
                }
              }
            }
            frame False {
              # "END NOT Found"
              n62 = Unbundle By Name(w159) -> ("Score"=w158:u32)
              n63 = Greater?(x=w158, y=w156) -> (0:w157:bool)
              n64 = case shown="False" w157 {
                tunnel: w162 -> [w165 w166]
                tunnel: [w164 w166] -> w160
                tunnel: w159 -> [w163 _]
                frame False {
                  n65 = Build Array (concatenate)(w165, w163) -> (w164:T1[])
                }
                frame True {
                  # "Score is Above Target Score"
                }
              }
            }
          }
        }
      }
    }
    n66 = Sort 1D Array(array=w68) -> (sorted array=w63:T1[])
    "sorted array" <- w63
    n67 = Array Size(array=w63) -> (size(s)=w62:i32)
    "size(s)" <- w62
    n68 = Less Or Equal To 0?(x=w62) -> (x <= 0?=w61:bool)
  }
  n69 = Collection Size(1:w5) -> (0:→"Answer":i32)
